vi "Copy Message Template.vi"(4 "Message Paths":T1, 7 "App":refnum<vi>, 8 "error in (no error)":errorcluster, 11 "LV-Protoc in":refnum<class "LV-Protoc.lvclass">) -> (0 "error out":errorcluster, 1 "Nested Libraries":refnum<vi>[](array[refnum]), 2 "VIs":refnum<vi>[](array[refnum]), 3 "LV-Protoc out":refnum<class "LV-Protoc.lvclass">, 5 "Library":refnum<vi>)   [LabVIEW 2020, in "LV-Protoc.lvlib" / "LV-Protoc.lvclass"]
uses:
  LV-Protoc.lvclass
  Message Paths.ctl
  LV-Protoc.lvlib
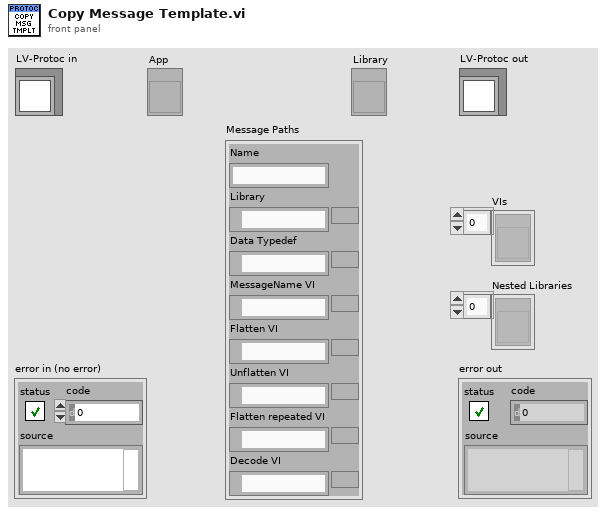
[diagram p1: front panel]
types:
  T1 = typedef "LV-Protoc.lvlib/Message Paths.ctl" = cluster{"Name":string, "Library":path, "Data Typedef":path, "MessageName VI":path, "Flatten VI":path, "Unflatten VI":path, "Flatten repeated VI":path, "Decode VI":path}
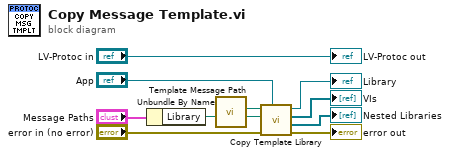
[diagram p0: block diagram]
diagram:
  n1 = Unbundle By Name("Message Paths") -> ("Library"=w10:path)
  n2 = call "Template Message Path.vi"() -> ("Template Library Path"=w8:path)  [unwired: 11 in]
  n3 = call "Copy Template Library.vi"("App"="App", "error in (no error)"="error in (no error)", "Destination lvlib Path"=w10, "Source lvlib Path"=w8) -> ("error out"=→"error out":errorcluster, "Nested Libraries"=→"Nested Libraries":refnum<vi>[], "VIs"=→"VIs":refnum<vi>[], "Library"=→"Library":refnum<vi>)  [unwired: 4 in]
  "LV-Protoc out" <- "LV-Protoc in"
